vi "Mosi Logic 256-bit.vi"(0 "data to send":bool[](array[boolean]), 5 "transfer settings":T2 {"Direction Change Bit" max=64 step=1; "Transfer Length (bits)" min=1 max=64 step=1}, 7 "controller interface":T1, 9 "shift MOSI":bool) -> (4 "MOSI":bool, 6 "MOSI enable":bool)   [LabVIEW 2015, in "SPI API.lvlib"]
doc: "This VI controls shifting MOSI data out of the FPGA."
uses:
  <userlib>/_NI SPI IP/FPGA/Controllers/Public/Transfer Settings.ctl
  Controls/Controller Interface.ctl
  SPI API.lvlib
  <userlib>/_NI SPI IP/FPGA/Controllers/NI SPI IP FPGA.lvlib
panel:
  # "This VI controls shifting MOSI data out of the FPGA."
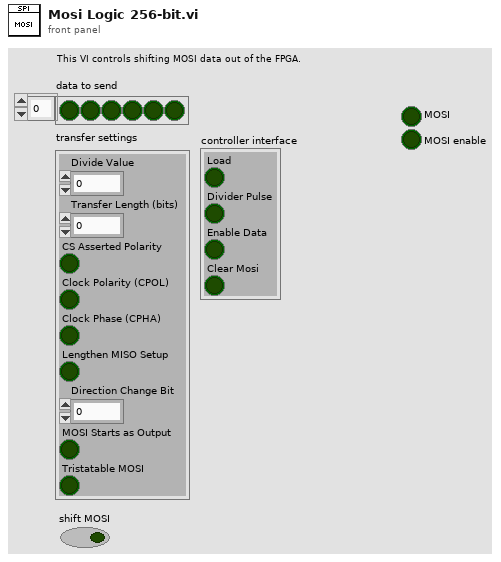
[diagram p1: front panel]
types:
  T1 = typedef "SPI API.lvlib/Controller Interface.ctl" = cluster{"Load":bool, "Divider Pulse":bool, "Enable Data":bool, "Clear Mosi":bool}
  T2 = typedef "NI SPI IP FPGA.lvlib/Transfer Settings.ctl" = cluster{"Divide Value":u8, "Transfer Length (bits)":u8, "CS Asserted Polarity":bool, "Clock Polarity (CPOL)":bool, "Clock Phase (CPHA)":bool, "Lengthen MISO Setup":bool, "Direction Change Bit":u8, "MOSI Starts as Output":bool, "Tristatable MOSI":bool}
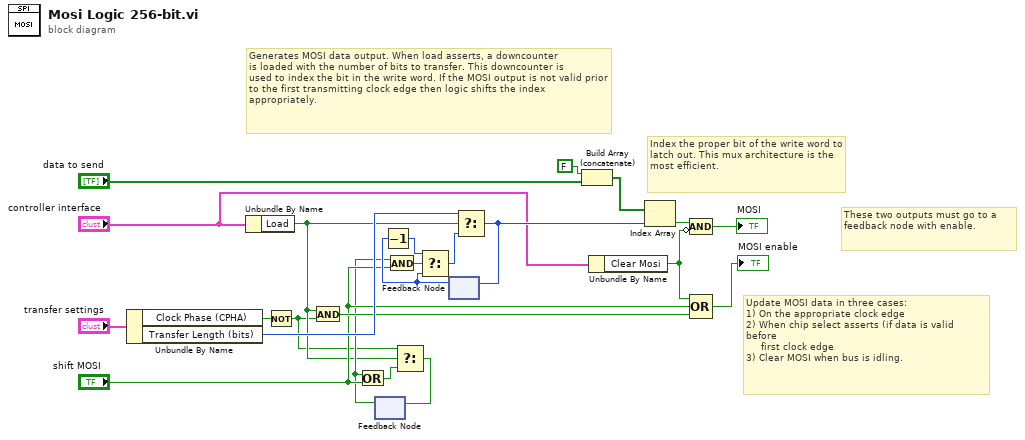
[diagram p0: block diagram]
diagram:
  # "These two outputs must go to a feedback node with enable."
  # "Generates MOSI data output. When load asserts, a downcounter\nis loaded with the number of bits to transfer. This downcounter is\nused to index the bit in the write word. If the MOSI output is not valid prior to the first transmitting clock edge then logic shifts the index appropriately."
  # "Update MOSI data in three cases:\n1) On the appropriate clock edge\n2) When chip select asserts (if data is valid before\n     first clock edge\n3) Clear MOSI when bus is idling."
  # "Index the proper bit of the write word to latch out. This mux architecture is the most efficient."
  n1 = Unbundle By Name("transfer settings") -> ("Clock Phase (CPHA)"=w6:bool, "Transfer Length (bits)"=w14:u8)
  n2 = Unbundle By Name("controller interface") -> ("Load"=w7:bool)
  n3 = Not(x=w6) -> (.not. x?=w5:bool)
  n4 = And(x=w7, y=w5) -> (x .and. y?=w13:bool)
  n5 = feedback #1() -> (w9:bool)  [unwired: 1 in]
  n6 = Or(x=w9, y="shift MOSI") -> (x .or. y?=w12:bool)
  n7 = And(x=w9, y="shift MOSI") -> (x .and. y?=w8:bool)
  n8 = Select(t=w5, s=w7, f=w12) -> (s? t:f=w11:bool)
  n9 = feedback-in #1(w11) -> ()
  n10 = feedback #2() -> (w21:u8)  [unwired: 1 in]
  n11 = Decrement(x=w21) -> (x-1=w23:u8)
  n12 = Select(t=w23, s=w8, f=w21) -> (s? t:f=w22:u8)
  n13 = Select(t=w14, s=w7, f=w22) -> (s? t:f=w18:u8)
  n14 = feedback-in #2(w18) -> ()
  n15 = Build Array (concatenate)(FALSE, "data to send") -> (w17:bool[])
  n16 = Unbundle By Name("controller interface") -> ("Clear Mosi"=w16:bool)
  n17 = Index Array(array=w17, index=w18) -> (element=w20:bool)
  n18 = Compound Arithmetic op=AND(w20, invert w16) -> (→"MOSI":bool)
  n19 = Compound Arithmetic op=OR(w16, "shift MOSI", w13) -> (→"MOSI enable":bool)
